vi "IncrementASCIITable.vi"(9 "0255array":u8[](array[numeric]), 10 "Numeric":i32, 11 "Array in":i32[](array[numeric])) -> (2 "we array":i32[](array[numeric]), 3 "Array out":i32[](array[numeric]))   [LabVIEW 2013]
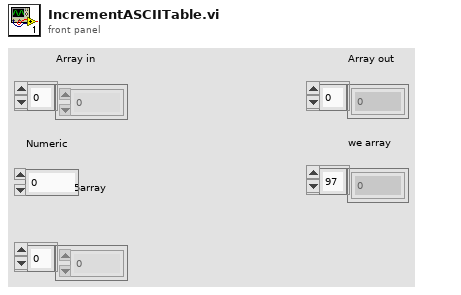
[diagram p1: front panel]
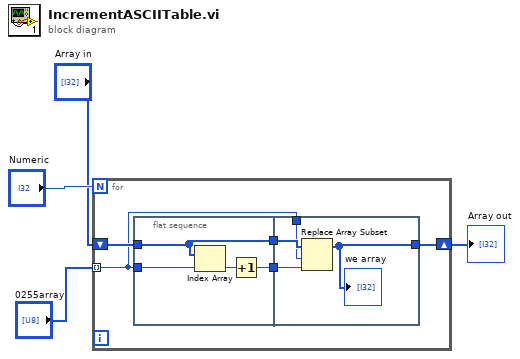
[diagram p0: block diagram]
diagram:
  n1 = for {
    N: "Numeric" -> [_]
    tunnel: "0255array" -> [w5] mode=indexing
    shift-right: [w6] -> w1
    shift-left: "Array in" -> [w9]
    n2 = flat-sequence {
      tunnel: w9 -> [w12]
      tunnel: w5 -> [w10]
      tunnel: [w12] -> w8
      tunnel: [w11] -> w7
      tunnel: w8 -> [w17]
      tunnel: w7 -> [w16]
      tunnel: [w15] -> w6
      tunnel: w5 -> [w14]
      frame #0 {
        n3 = Index Array(array=w12, index=w10) -> (element=w13:i32)
        n4 = Increment(x=w13) -> (x+1=w11:i32)
      }
      frame #1 {
        n5 = Replace Array Subset(array=w17, new element=w16, index=w14) -> (w15:i32[])
        "we array" <- w15
      }
    }
  }
  "Array out" <- w1
